vi "load waveforms_tt.vi"(1 "waveform":path) -> (0 "# of points":i32)   [LabVIEW 2013]
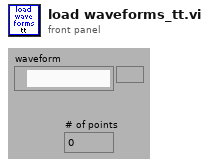
[diagram p1: front panel]
types:
  T1 = cluster{"Xpixels":i32, "Vx-min ref":dbl, "Vx-max ref":dbl, "Ypixels":i32, "Vy-min ref":dbl, "Vy-max ref":dbl, "srate":dbl, "type":string, "date":string, "time":string, "Colormap":u16, "square pixels":bool, "square matrix":bool, "Xpixels Img":i32, "Vx-min Img":dbl, "VX-max Img":dbl, "Ypixels Img":i32, "Vy-min Img":dbl, "Vy-max Img ":dbl, "autoshutter":bool, "P":dbl, "sAOxy":i32, "finite":bool, "cont":bool, "wavdet":bool, "measpoints":i32, "avpp":i32, "bufferAO":i32, "bufferAI":i32, "CH1":bool, "CH2":bool, "X":bool, "Y":bool, "timeout":dbl, "starttick":u32, "waveform":path, "Vy-ref":dbl, "Vx-ref":dbl, "refreshrate":dbl, "refreshbuffer":i32, "tt_cycles":i32, "motorref":refnum<k7>, "mirrorswitch":refnum<k7>, "sample mode":i32}
  T2 = cluster{"VtoP":dbl[], "CWlasers":dbl[], "shutter":dbl[], "488":dbl[], "532":dbl[], "640":dbl[]}
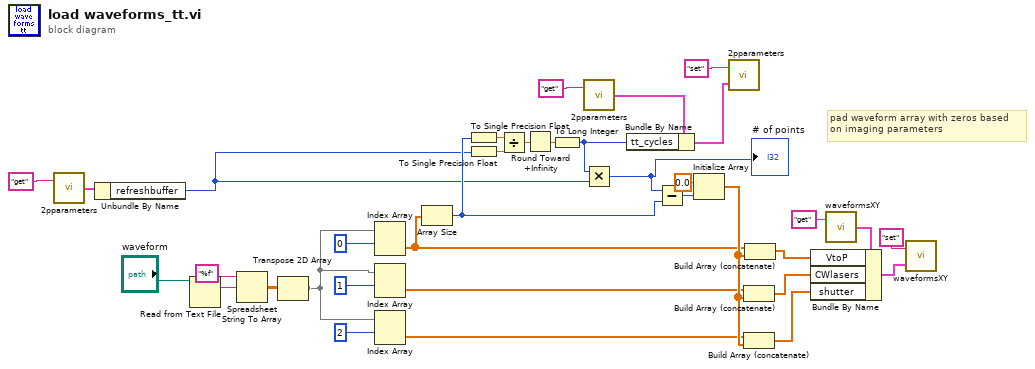
[diagram p0: block diagram]
diagram:
  # "pad waveform array with zeros based\non imaging parameters"
  n1 = call "2pparameters.vi"("command"="get") -> ("Params out"=w18:T1)  [unwired: 1 in]
  n2 = Unbundle By Name(w18) -> ("refreshbuffer"=w7:i32)
  n3 = Read from Text File(file (use dialog)="waveform") -> (text=w16:string)  [unwired: 3 in, 3 out]
  n4 = Spreadsheet String To Array(format string="%f", spreadsheet string=w16) -> (array=w14:dbl[][])  [unwired: 2 in]
  n5 = Transpose 2D Array(2D array=w14) -> (transposed array=w10:dbl[][])
  n6 = Index Array(array=w10, index (row)=0) -> (element=w29:dbl[])  [unwired: 1 in]
  n7 = Index Array(array=w10, index (row)=1) -> (element=w30:dbl[])  [unwired: 1 in]
  n8 = Index Array(array=w10, index (row)=2) -> (element=w31:dbl[])  [unwired: 1 in]
  n9 = Array Size(array=w29) -> (size(s)=w9:i32)
  n10 = To Single Precision Float(number=w9) -> (single precision float=w19:sgl)
  n11 = To Single Precision Float(number=w7) -> (single precision float=w20:sgl)
  n12 = Divide(x=w19, y=w20) -> (x/y=w21:sgl)
  n13 = Round Toward +Infinity(x=w21) -> (ceil(x): smallest int >= x=w22:sgl)
  n14 = To Long Integer(number=w22) -> (32bit integer=w2:i32)
  n15 = call "2pparameters.vi"("command"="get") -> ("Params out"=w5:T1)  [unwired: 1 in]
  n16 = Multiply(x=w2, y=w7) -> (x*y=w1:i32)
  "# of points" <- w1
  n17 = Bundle By Name(cluster=w5, "tt_cycles"=w2) -> (w3:T1)
  n18 = Subtract(x=w1, y=w9) -> (x-y=w27:i32)
  n19 = Initialize Array(0.0 ("element"), w27) -> (w32:dbl[])
  n20 = call "2pparameters.vi"("Params in"=w3, "command"="set") -> ()  [unwired: 1 out]
  n21 = Build Array (concatenate)(w30, w32) -> (w34:dbl[])
  n22 = Build Array (concatenate)(w31, w32) -> (w35:dbl[])
  n23 = Build Array (concatenate)(w29, w32) -> (w33:dbl[])
  n24 = call "waveformsXY.vi"("command"="get") -> ("waveforms out"=w24:T2)  [unwired: 1 in]
  n25 = Bundle By Name(cluster=w24, "VtoP"=w33, "CWlasers"=w34, "shutter"=w35) -> (w26:T2)
  n26 = call "waveformsXY.vi"("waveforms in"=w26, "command"="set") -> ()  [unwired: 1 out]
